vi "Control Init.vi"(7 "VolatusAPI":refnum<class "VolatusAPI.lvclass">, 8 "error in (no error)":errorcluster, 10 "JSON":string, 11 "ButtonControl in":refnum<class "DigitalButtonControl.lvclass">) -> (0 "error out":errorcluster, 3 "ButtonControl out":refnum<class "DigitalButtonControl.lvclass">)   [LabVIEW 2020, in "VolatusGUIElements.lvlib" / "DigitalButtonControl.lvclass"]
uses:
  DigitalButtonControl.lvclass
  DigitalButtonControl.lvclass/DigitalButtonControl.ctl
  7f1ddf9b-cd10-40fa-bddf-b675369dd94f.vi
  VolatusGUI/GUI Element/GUI Element.lvclass
  Volatus/VolatusAPI/VolatusAPI.lvclass
  lv-vecto/Vecto/Group/Group.lvclass
  VolatusGUIElements.lvlib
  C:/dev/lv20CE/relink/lv-volatus/VolatusGUI/Control/Control.lvclass
  C:/dev/lv20CE/relink/lv-volatus/VolatusGUI/GUI Element/GUI Element.lvclass
  C:/dev/lv20CE/relink/lv-volatus/VolatusGUIElements/DigitalButtonControl/DigitalButtonControl.lvclass
  C:/dev/lv20CE/relink/lv-volatus/VolatusGUI/OnValueChangeHandler/OnValueChangeHandler.lvclass
  C:/dev/lv20CE/relink/lv-vecto/Vecto/GroupAbstract/GroupAbstract.lvclass
  C:/dev/lv20CE/relink/lv-vecto/Vecto/Group/Group.lvclass
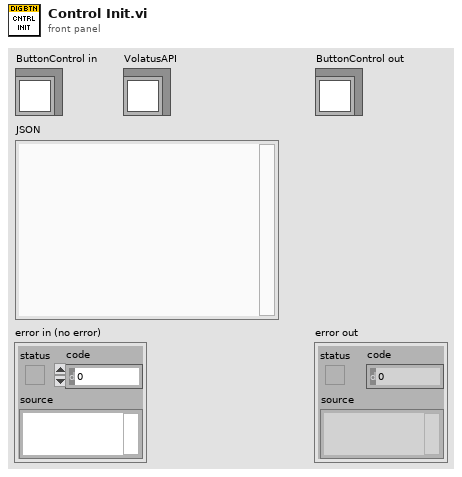
[diagram p1: front panel]
types:
  T1 = typedef "VolatusGUIElements.lvlib/DigitalButtonControl.lvclass/JSON.ctl" = cluster{"Node":string, "Task":string, "Group":string, "Channel":string, "Invert":bool, "Staleness":dbl, "Appearance":cluster{"TextColor":string, "Unclicked":T2, "Clicked":T2}}
  T2 = typedef "VolatusGUIElements.lvlib/DigitalButtonControl.lvclass/Appearance.ctl" = cluster{"Text":string, "Color":string}
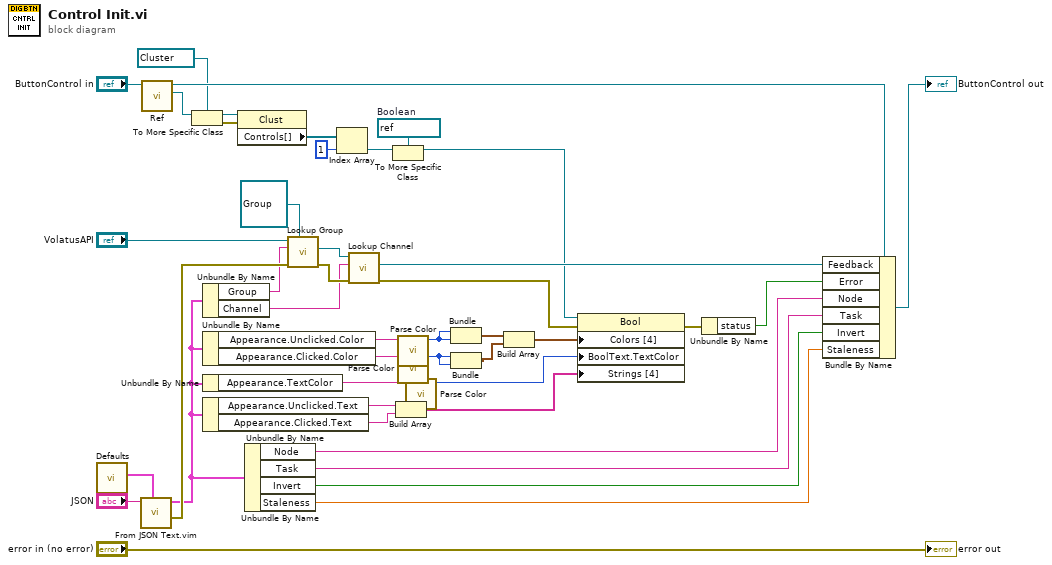
[diagram p0: block diagram]
diagram:
  w27 = refnum<vi> refnum  # Boolean
  n1 = call "Defaults.vi"() -> ("Defaults"=w22:T1)  [unwired: 11 in]
  n2 = call "From JSON Text.vim"("Data Type and Default Value"=w22, "JSON"="JSON") -> ("error out"=w43:errorcluster, "Data out"=w5:T1)  [unwired: 8 in]
  n3 = call "Ref.vi"("GUI Element in"="ButtonControl in") -> ("Ref"=w39:refnum<vi>, "GUI Element out"=w40:refnum<class "DigitalButtonControl.lvclass">)  [unwired: 9 in]
  n4 = To More Specific Class(target class=refnum<vi> refnum ("specific class reference"), reference=w39) -> (specific class reference=w37:refnum<vi>, error out=w36:errorcluster)  [unwired: 1 in]
  n5 = Unbundle By Name(w5) -> ("Group"=w34:string, "Channel"=w30:string)
  n6 = Unbundle By Name(w5) -> ("Appearance.Unclicked.Color"=w21:string, "Appearance.Clicked.Color"=w20:string)
  n7 = Unbundle By Name(w5) -> ("Appearance.TextColor"=w19:string)
  n8 = Unbundle By Name(w5) -> ("Appearance.Unclicked.Text"=w18:string, "Appearance.Clicked.Text"=w17:string)
  n9 = property class="Clust"(reference=w37, error in=w36) -> ("Controls[]"=w26:refnum<vi>[])  [unwired: 2 out]
  n10 = Unbundle By Name(w5) -> ("Node"=w4:string, "Task"=w3:string, "Invert"=w2:bool, "Staleness"=w1:dbl)
  n11 = call "Lookup Group.vi"("Group Type (Abstract)"=refnum<class "Group.lvclass"> refnum ("Vecto.lvlib:Group.lvclass"), "error in (no error)"=w43, "Group Name"=w34, "VolatusAPI in"="VolatusAPI") -> ("error out"=w31:errorcluster, "Group"=w32:refnum<class "Group.lvclass">)  [unwired: 5 in, 1 out]
  n12 = Index Array(array=w26, index=1) -> (element=w24:refnum<vi>)
  n13 = call "Lookup Channel.vi"("error in (no error)"=w31, "Channel Name"=w30, "Group in"=w32) -> ("error out"=w9:errorcluster, "Channel"=w28:refnum<class "Channel.lvclass">)  [unwired: 6 in, 1 out]
  n14 = To More Specific Class(target class=w27, reference=w24) -> (specific class reference=w23:refnum<vi>)  [unwired: 1 in, 1 out]
  n15 = Build Array(w18, w17) -> (w10:string[])
  n16 = call "Parse Color.vi"("Color String"=w21) -> ("Color"=w15:u32)  [unwired: 9 in, 1 out]
  n17 = call "Parse Color.vi"("Color String"=w20) -> ("Color"=w14:u32)  [unwired: 9 in, 1 out]
  n18 = call "Parse Color.vi"("Color String"=w19) -> ("Color"=w16:u32)  [unwired: 9 in, 1 out]
  n19 = Bundle("Color"=w15, "Color"=w15) -> (w13:cluster{"Color":u32, "Color":u32})  [unwired: 1 in]
  n20 = Bundle("Color"=w14, "Color"=w14) -> (w12:cluster{"Color":u32, "Color":u32})  [unwired: 1 in]
  n21 = Build Array(w13, w12) -> (w11:cluster{"Color":u32, "Color":u32}[])
  n22 = property class="Bool"(reference=w23, error in=w9, "Colors [4]"=w11, "BoolText.TextColor"=w16, "Strings [4]"=w10) -> (error out=w8:errorcluster)  [unwired: 1 out]
  n23 = Unbundle By Name(w8) -> ("status"=w6:bool)
  n24 = Bundle By Name(cluster=w40, "Feedback"=w28, "Error"=w6, "Node"=w4, "Task"=w3, "Invert"=w2, "Staleness"=w1) -> (→"ButtonControl out":refnum<class "DigitalButtonControl.lvclass">)
  "error out" <- "error in (no error)"
